vi "_PathQ.vi"(8 "error in (no error)":errorcluster) -> (0 "error out":errorcluster, 3 "Queue out":refnum<queue>)   [LabVIEW 2019, in "LabVIEW-VIProviderShell.lvlib" / "VIProviderShellHelper.lvclass"]
uses:
  VIProviderShellHelper.lvclass
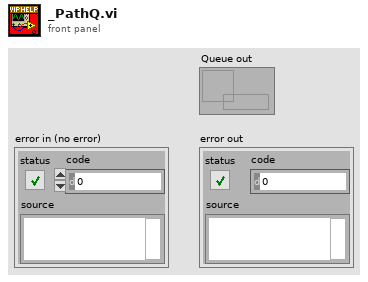
[diagram p1: front panel]
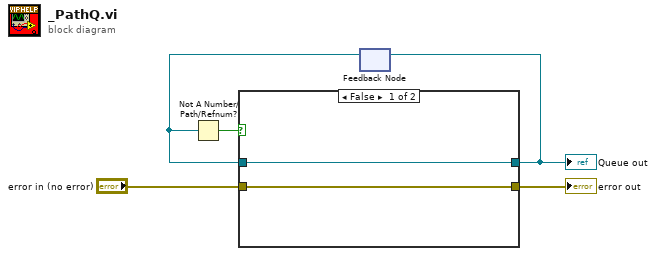
[diagram p0: block diagram]
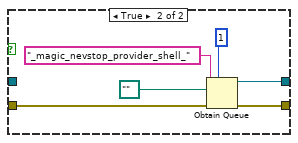
[diagram p2: hidden frame]
diagram:
  n1 = feedback #1() -> (w2:refnum<queue>)  [unwired: 1 in]
  n2 = Not A Number/Path/Refnum?(number/path/refnum=w2) -> (NaN/Path/Refnum?=w1:bool)
  n3 = case shown="False" w1 {
    tunnel: [w6 w13] -> w3
    tunnel: [w7 w12] -> w5
    tunnel: "error in (no error)" -> [w6 w9]
    tunnel: w2 -> [w7 _]
    frame False {
    }
    frame True {
      n4 = Obtain Queue(max queue size (-1, unlimited)=1, name (unnamed)="_magic_nevstop_provider_shell_", element data type=path "" ("Initialize-API"), error in (no error)=w9) -> (queue out=w12:refnum<queue>, error out=w13:errorcluster)  [unwired: 1 in, 1 out]
    }
  }
  "Queue out" <- w5
  "error out" <- w3
  n5 = feedback-in #1(w5) -> ()
